vi "percent true of DeviationArray.vi"(2 "DeviationArray":cluster{"X Centroid":sgl, "Y Centroid":sgl}[](array[cluster]), 3 "Threshold":cluster{"X Target":sgl, "Y Target":sgl}={"X Target"=279.44305, "Y Target"=323.3971}) -> (7 "% XY State True":cluster{dbl, dbl})   [LabVIEW 2013]
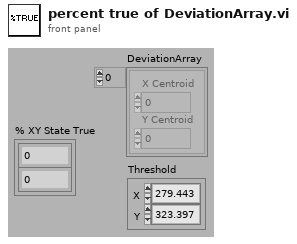
[diagram p1: front panel]
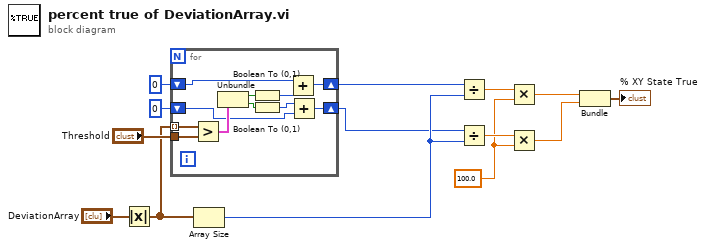
[diagram p0: block diagram]
diagram:
  w12 = 100.0 ("y")
  n1 = Absolute Value(x="DeviationArray") -> (abs(x)=w1:cluster{"X Centroid":sgl, "Y Centroid":sgl}[])
  n2 = for {
    tunnel: w1 -> [w25] mode=indexing
    tunnel: "Threshold" -> [w24]
    shift-right: [w17] -> w2
    shift-left: i16 0 -> [w15]
    shift-right: [w19] -> w4
    shift-left: i16 0 -> [w18]
    n3 = Greater?(x=w25, y=w24) -> (0:w23:cluster{bool, bool})
    n4 = Unbundle(w23) -> (w22:bool, w20:bool)
    n5 = Boolean To (0,1)(Boolean=w22) -> (0, 1=w21:i16)
    n6 = Boolean To (0,1)(Boolean=w20) -> (0, 1=w16:i16)
    n7 = Add(x=w18, y=w21) -> (x+y=w19:i16)
    n8 = Add(x=w16, y=w15) -> (x+y=w17:i16)
  }
  n9 = Array Size(array=w1) -> (size(s)=w3:i32)
  n10 = Divide(x=w4, y=w3) -> (x/y=w13:dbl)
  n11 = Divide(x=w2, y=w3) -> (x/y=w14:dbl)
  n12 = Multiply(x=w13, y=w12) -> (x*y=w11:dbl)
  n13 = Multiply(x=w14, y=w12) -> (x*y=w10:dbl)
  n14 = Bundle(w11, w10) -> (→"% XY State True":cluster{dbl, dbl})  [unwired: 1 out]
